vi "keithly set-up_VISA.vi"(8 "error in":errorcluster, 10 "ConfigOpt":i16(ring)=1 items=["SAV0", "SAV1", "SAV2", "SAV3", "SAV4", "SAV5", "SAV6", "SAV7", "SAV8", "SAV9", "RST", "Preset"]) -> (0 "error out":errorcluster, 3 "meter-VISA":refnum<visa-resource-name>)   [LabVIEW 2024]
doc: "VI intializes connection to Keithley 6517 picoampmeter (K6517) to read photodiode currents for reflectivity test station.\n\nK6517 must be connected to to PC via GPIB."
uses:
  <instrlib>/Keithley 6517/Keithley 6517.lvlib
panel:
  # "Start Keithley 6517 Electrometer"
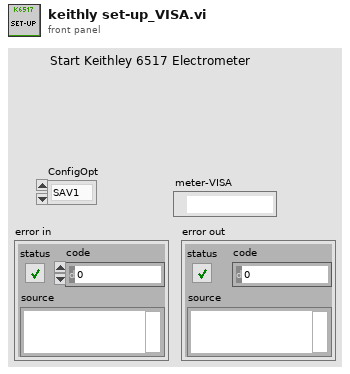
[diagram p1: front panel]
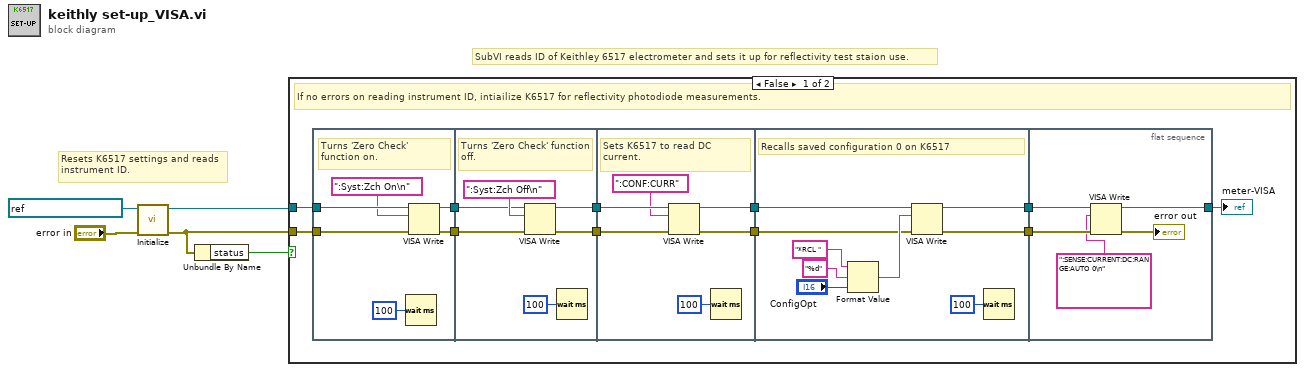
[diagram p0: block diagram]
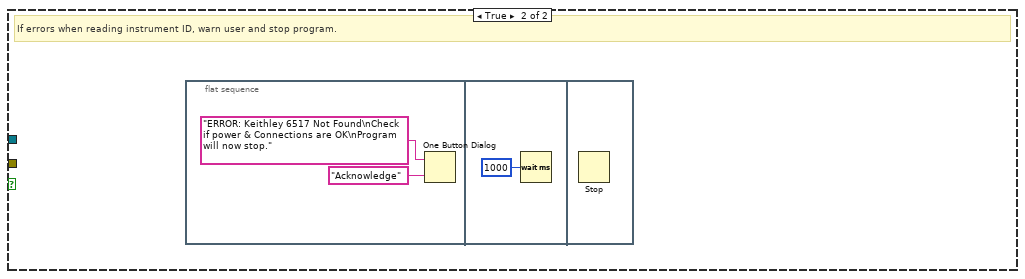
[diagram p2: hidden frame]
diagram:
  # "Resets K6517 settings and reads\ninstrument ID."
  # "SubVI reads ID of Keithley 6517 electrometer and sets it up for reflectivity test staion use."
  n1 = call <instrlib>:"Initialize.vi"("error in (no error)"="error in", "VISA resource name"=refnum<visa-resource-name> "GPIB0::27::INSTR") -> ("error out"=w4:errorcluster, "VISA resource name out"=w1:refnum<visa-resource-name>)  [unwired: 8 in]
  n2 = Unbundle By Name(w4) -> ("status"=w5:bool)
  n3 = case shown="False" w5 {
    tunnel: w4 -> [w14 _]
    tunnel: w1 -> [w12 _]
    frame False {
      # "If no errors on reading instrument ID, intiailize K6517 for reflectivity photodiode measurements."
      n4 = flat-sequence {
        tunnel: w14 -> [w21]
        tunnel: [w20] -> w16
        tunnel: w12 -> [w19]
        tunnel: [w17] -> w11
        tunnel: w16 -> [w27]
        tunnel: [w26] -> w15
        tunnel: w11 -> [w24]
        tunnel: [w23] -> w10
        tunnel: w15 -> [w32]
        tunnel: w10 -> [w33]
        tunnel: [w30] -> w9
        tunnel: [w29] -> w8
        tunnel: [w36] -> w13
        tunnel: w9 -> [w42]
        tunnel: w8 -> [w37]
        tunnel: [w35] -> w7
        tunnel: w13 -> [w48]
        tunnel: w7 -> [w45]
        tunnel: [w44] -> w6
        frame #0 {
          # "Turns 'Zero Check' function on."
          n5 = Wait (ms)(milliseconds to wait=u32 100) -> ()  [unwired: 1 out]
          n6 = VISA Write(VISA resource name=w19, write buffer=":Syst:Zch On\n", error in (no error)=w21) -> (VISA resource name out=w17:refnum<visa-resource-name>, error out=w20:errorcluster)  [unwired: 1 out]
        }
        frame #1 {
          # "Turns 'Zero Check' function off."
          n7 = VISA Write(VISA resource name=w24, write buffer=":Syst:Zch Off\n", error in (no error)=w27) -> (VISA resource name out=w23:refnum<visa-resource-name>, error out=w26:errorcluster)  [unwired: 1 out]
          n8 = Wait (ms)(milliseconds to wait=u32 100) -> ()  [unwired: 1 out]
        }
        frame #2 {
          # "Sets K6517 to read DC current."
          n9 = VISA Write(VISA resource name=w33, write buffer=":CONF:CURR", error in (no error)=w32) -> (VISA resource name out=w30:refnum<visa-resource-name>, error out=w29:errorcluster)  [unwired: 1 out]
          n10 = Wait (ms)(milliseconds to wait=u32 100) -> ()  [unwired: 1 out]
        }
        frame #3 {
          # "Recalls saved configuration 0 on K6517"
          n11 = Format Value(string ("")="*RCL ", format string="%d", value (0)="ConfigOpt") -> (output string=w38:string)
          n12 = VISA Write(VISA resource name=w42, write buffer=w38, error in (no error)=w37) -> (VISA resource name out=w35:refnum<visa-resource-name>, error out=w36:errorcluster)  [unwired: 1 out]
          n13 = Wait (ms)(milliseconds to wait=u32 100) -> ()  [unwired: 1 out]
        }
        frame #4 {
          n14 = VISA Write(VISA resource name=w45, write buffer=":SENSE:CURRENT:DC:RANGE:AUTO 0\n", error in (no error)=w48) -> (VISA resource name out=w44:refnum<visa-resource-name>, error out=→"error out":errorcluster)  [unwired: 1 out]
        }
      }
      "meter-VISA" <- w6
    }
    frame True {
      # "If errors when reading instrument ID, warn user and stop program."
      n15 = flat-sequence {
        frame #0 {
          n16 = One Button Dialog(message="ERROR: Keithley 6517 Not Found\nCheck if power & Connections are OK\nProgram will now stop.", button name ("OK")="Acknowledge") -> ()  [unwired: 1 out]
        }
        frame #1 {
          n17 = Wait (ms)(milliseconds to wait=u32 1000) -> ()  [unwired: 1 out]
        }
        frame #2 {
          n18 = Stop() -> ()  [unwired: 1 in]
        }
      }
    }
  }
